vi "Revision Query.vi"(0 "VISA resource name":refnum<visa-resource-name>, 11 "error in (no error)":errorcluster) -> (4 "VISA resource name out":refnum<visa-resource-name>, 8 "Instr Driver Revision":string, 10 "Instr Firmware Revision":string, 15 "error out":errorcluster)   [LabVIEW 2020, in "Yokogawa WT200 Series.lvlib"]
doc: "This VI queries the current instrument firmware revision and instrument driver revision.\n\nThis Instrument Driver's Revision number is 1.10 and is compatible with Instrument Firmware Revision F3.11(WT200), F1.06(WT210/WT230)\n\nYOKOGAWA WT200/WT210/WT230 Digital Power Meter\nCreated By: Yokogawa Electric Corporation\nRelease Date: 09/2002\nOriginally Developed in LabVIEW Version: 5.0.1\n\nModification History: \n\n1.10 09/2002 Add support instrument WT210 and WT230.\n Add support serial interface.\n Add YKWT230 Config Wiring.vi, YKWT200 Config Sample Rate.vi, YKWT200 Read Measure Binary.vi, YKWT200 Remote.vi."
uses:
  Yokogawa WT200 Series.lvlib
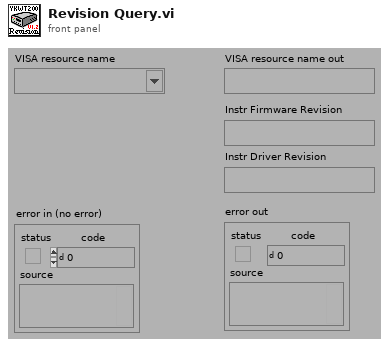
[diagram p1: front panel]
types:
  T1 = enum32{"invalid app kind", "Development System", "Run Time System", "Student Edition", "Embedded LabVIEW", "Evaluation", "Custom"}
  T2 = cluster{"Major":u16, "Minor":u16, "Fix":u16, "Build":u16}
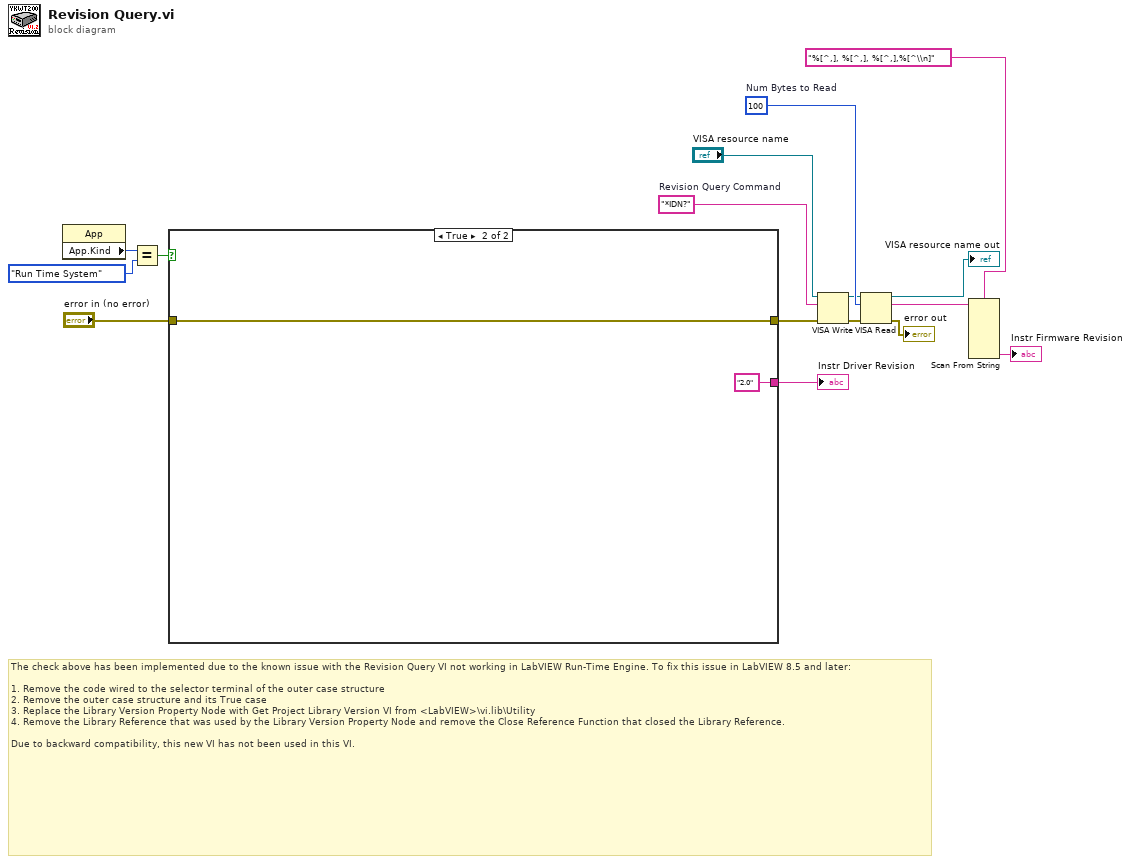
[diagram p0: block diagram]
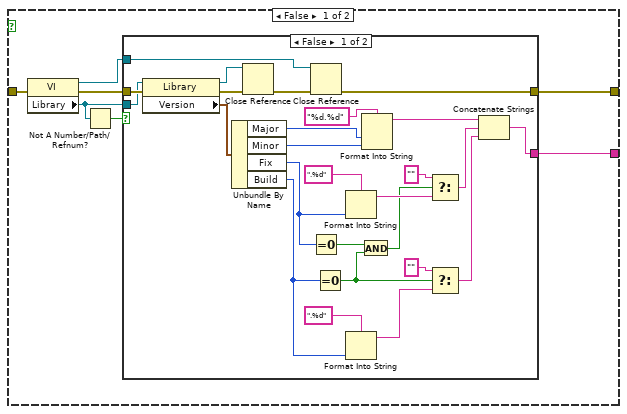
[diagram p2: hidden frame]
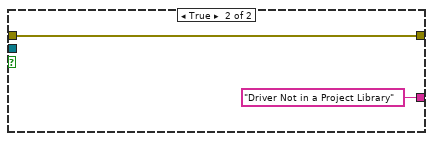
[diagram p3: hidden frame]
diagram:
  w13 = "*IDN?"  # Revision Query Command
  w16 = u32 100  # Num Bytes to Read
  # "The check above has been implemented due to the known issue with the Revision Query VI not working in LabVIEW Run-Time Engine. To fix this issue in LabVIEW 8.5 and later:\n\n1. Remove the code wired to the selector terminal of the outer case structure\n2. Remove the outer case structure and its True case\n3. Replace the Library Version Property Node with Get Project Library Version VI from <LabVIEW>\\vi.lib\\Utility\n4. Remove the Library Reference that was used by the Library Version Property Node and remove the Close Reference Function that closed the Library Reference.\n\nDue to backward compatibility, this new VI has not been used in this VI."
  n1 = property class="App"() -> ("App.Kind"=w2:T1)  [unwired: 2 in, 2 out]
  n2 = Equal?(x=w2, y=T1."Run Time System") -> (x = y?=w3:bool)
  n3 = case shown="True" w3 {
    tunnel: "error in (no error)" -> [w23 w53]
    tunnel: [w18 "2.0"] -> w5
    tunnel: [w17 w53] -> w4
    frame False {
      n4 = property class="VI"(error in=w23) -> (reference out=w19:refnum<vi>, error out=w22:errorcluster, "Library"=w21:refnum<vi>)  [unwired: 1 in]
      n5 = Not A Number/Path/Refnum?(number/path/refnum=w21) -> (NaN/Path/Refnum?=w20:bool)
      n6 = case shown="False" w20 {
        tunnel: [w28 w50] -> w17
        tunnel: [w27 "Driver Not in a Project Library"] -> w18
        tunnel: w22 -> [w26 w50]
        tunnel: w21 -> [w25 _]
        tunnel: w19 -> [w24 _]
        frame False {
          n7 = property class="Library"(reference=w25, error in=w26) -> (reference out=w48:refnum<vi>, error out=w49:errorcluster, "Version"=w46:T2)
          n8 = Unbundle By Name(w46) -> ("Major"=w35:u16, "Minor"=w34:u16, "Fix"=w32:u16, "Build"=w33:u16)
          n9 = Close Reference(reference=w48, error in (no error)=w49) -> (error out=w47:errorcluster)
          n10 = Close Reference(reference=w24, error in (no error)=w47) -> (error out=w28:errorcluster)
          n11 = Equal To 0?(x=w32) -> (x = 0?=w31:bool)
          n12 = Equal To 0?(x=w33) -> (x = 0?=w30:bool)
          n13 = Format Into String(format string=".%d", w32) -> (resulting string=w43:string)  [unwired: 2 in, 1 out]
          n14 = Format Into String(format string=".%d", w33) -> (resulting string=w39:string)  [unwired: 2 in, 1 out]
          n15 = And(x=w31, y=w30) -> (x .and. y?=w29:bool)
          n16 = Format Into String(format string="%d.%d", w35, w34) -> (resulting string=w41:string)  [unwired: 2 in, 1 out]
          n17 = Select(t="", s=w29, f=w43) -> (s? t:f=w40:string)
          n18 = Select(t="", s=w30, f=w39) -> (s? t:f=w36:string)
          n19 = Concatenate Strings(w41, w40, w36) -> (w27:string)
        }
        frame True {
        }
      }
    }
    frame True {
    }
  }
  "Instr Driver Revision" <- w5
  n20 = VISA Write(VISA resource name="VISA resource name", write buffer=w13, error in (no error)=w4) -> (VISA resource name out=w15:refnum<visa-resource-name>, error out=w14:errorcluster)  [unwired: 1 out]
  n21 = VISA Read(VISA resource name=w15, byte count=w16, error in (no error)=w14) -> (VISA resource name out=→"VISA resource name out":refnum<visa-resource-name>, read buffer=w12:string, error out=→"error out":errorcluster)  [unwired: 1 out]
  n22 = Scan From String(format string="%[^,], %[^,], %[^,],%[^\\n]", input string=w12) -> (output 4=→"Instr Firmware Revision":string)  [unwired: 9 in, 3 out]
